vi "Generate_SN.vi"(8 "error in (no error)":errorcluster caption="entrée d'erreur (pas d'erreur)", 11 "Class Creation_SN (Default) en entrée":refnum<class "Creation_SN_Nodon.lvclass">) -> (0 "error out":errorcluster caption="sortie d'erreur", 3 "Class Creation_SN (Default) en sortie":refnum<class "Creation_SN_Nodon.lvclass">)   [LabVIEW 2020, in "Library Instrument & Equipement.lvlib" / "Library Creation_SN.lvlib" / "Creation_SN_Nodon.lvclass"]
uses:
  Creation_SN_Nodon.lvclass
  C:/Users/ngarcin/OneDrive - Altyor/Standard TB/Class/Creation_SN/Creation_SN Database (Default)/Creation_SN Database (Default).lvclass
  C:/Users/ngarcin/OneDrive - Altyor/Standard TB/Class/Creation_SN/Creation_SN (Default)/Creation_SN (Virtual).lvclass
  Creation_SN_Nodon.lvclass/Creation_SN_Nodon.ctl
  Creation_SN Database (Default)/Creation_SN Database (Default).lvclass
  Firebase/Source/Firebase Recovery_SN/Firebase Recovery_SN.lvclass
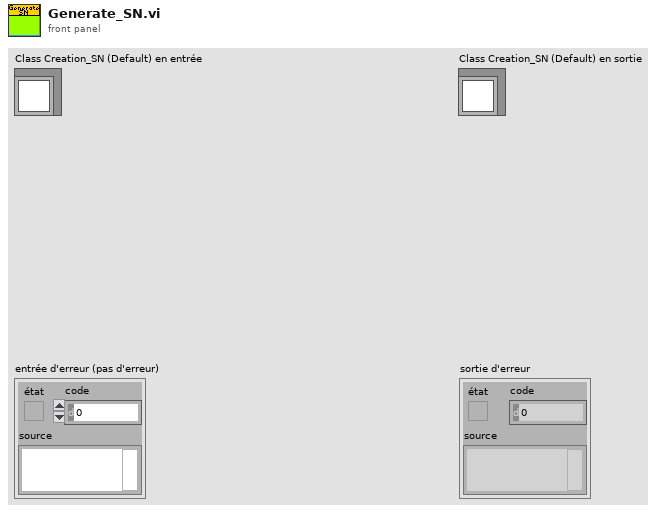
[diagram p1: front panel]
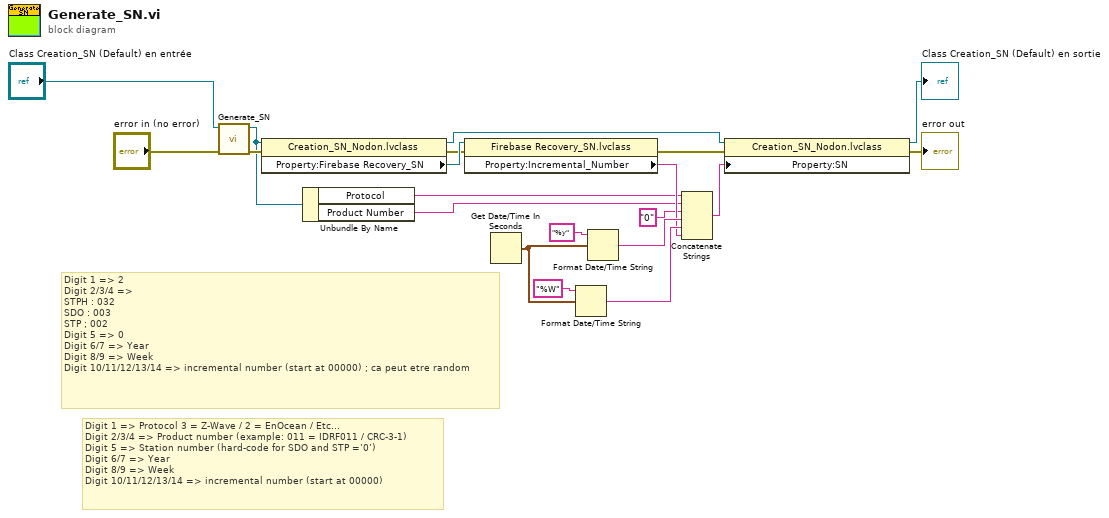
[diagram p0: block diagram]
diagram:
  # "Digit 1 => Protocol 3 = Z-Wave / 2 = EnOcean / Etc…\nDigit 2/3/4 => Product number (example: 011 = IDRF011 / CRC-3-1)\nDigit 5 => Station number (hard-code for SDO and STP =’0’)\nDigit 6/7 => Year\nDigit 8/9 => Week\nDigit 10/11/12/13/14 => incremental number (start at 00000)"
  # "Digit 1 => 2\nDigit 2/3/4 =>\nSTPH : 032\nSDO : 003\nSTP ; 002\nDigit 5 => 0\nDigit 6/7 => Year\nDigit 8/9 => Week\nDigit 10/11/12/13/14 => incremental number (start at 00000) ; ca peut etre random"
  n1 = call-parent "Generate_SN.vi"("error in (no error)"="error in (no error)", "Class Creation_SN (Default) en entrée"="Class Creation_SN (Default) en entrée") -> ("error out"=w11:errorcluster, "Class Creation_SN (Default) en sortie"=w4:refnum<class "Creation_SN_Nodon.lvclass">)  [unwired: 8 in]
  n2 = property class="Creation_SN_Nodon.lvclass"(reference=w4, error in=w11) -> (reference out=w9:refnum<class "Creation_SN_Nodon.lvclass">, error out=w10:errorcluster, "Property:Firebase Recovery_SN"=w12:refnum<class "Firebase Recovery_SN.lvclass">)
  n3 = Unbundle By Name(w4) -> ("Protocol"=w3:string, "Product Number"=w2:string)
  n4 = property class="Firebase Recovery_SN.lvclass"(reference=w12, error in=w10) -> (error out=w8:errorcluster, "Property:Incremental_Number"=w13:string)  [unwired: 1 out]
  n5 = Get Date/Time In Seconds() -> (seconds since 1Jan1904=w16:timestamp)
  n6 = Format Date/Time String(time format string (%c)="%W" ("chaîne de format de l'heure (%c)"), seconds (now)=w16) -> (date/time string=w14:string)  [unwired: 1 in]
  n7 = Format Date/Time String(time format string (%c)="%y" ("chaîne de format de l'heure (%c)"), seconds (now)=w16) -> (date/time string=w15:string)  [unwired: 1 in]
  n8 = Concatenate Strings(w3, w2, "0" ("élément"), w15, w14, w13) -> (w1:string)
  n9 = property class="Creation_SN_Nodon.lvclass"(reference=w9, error in=w8, "Property:SN"=w1) -> (reference out=→"Class Creation_SN (Default) en sortie":refnum<class "Creation_SN_Nodon.lvclass">, error out=→"error out":errorcluster)
